vi "DeviceDiscover.vi"(0 "GenericDevice in":refnum<class "GenericDevice.lvclass">, 1 "Delay between send and receive [ms]":i32=5000, 5 "error in (no error)":errorcluster) -> (14 "GenericDevice out":refnum<class "GenericDevice.lvclass">, 15 "count":i32, 16 "ID":i32, 17 "returned command":string, 18 "error string (if existing)":string, 19 "error out":errorcluster)   [LabVIEW 2023, in "GenericDevice.lvclass"]
uses:
  GenericDevice.lvclass
  Discover.ctl
  GenericDevice.lvclass/GenericDevice.ctl
  f3c4c4a7-1197-4301-b128-d95ffad61759.vi
  8dcdfc4e-e41c-41c3-8bf5-06d7d5a87ca3.vi
  7995de1f-19cd-413c-9dd1-d9467f03dc24.vi
  <vilib>/JDP Science/JSONtext/Variant to JSON Text.vi
  <vilib>/JDP Science/JSONtext/Set Item.vi
  <vilib>/JDP Science/JSONtext/JSON text to Variant.vi
  <vilib>/JDP Science/JSONtext/LVClass Serializer/JSONtext LVClass Serializer.lvclass
panel:
  # "Connector Pane"
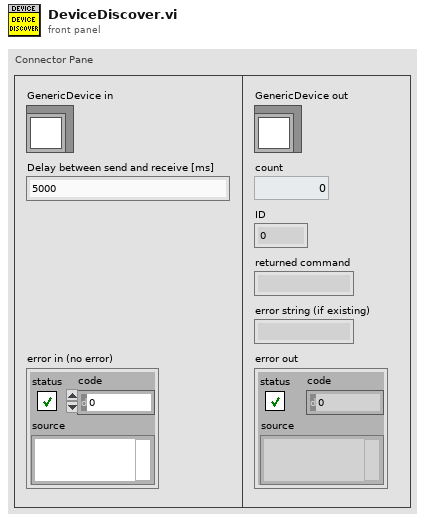
[diagram p1: front panel]
types:
  T1 = typedef "GenericDevice.lvclass/Discover.ctl" = cluster{"count":i32}
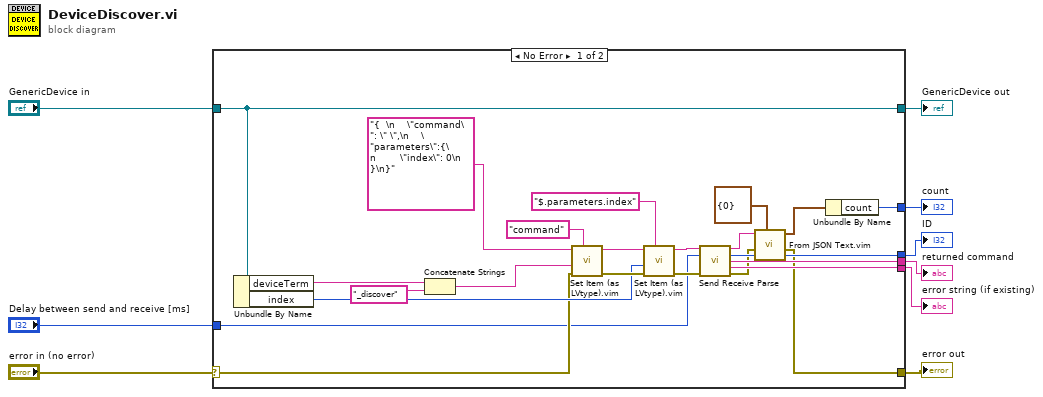
[diagram p0: block diagram]
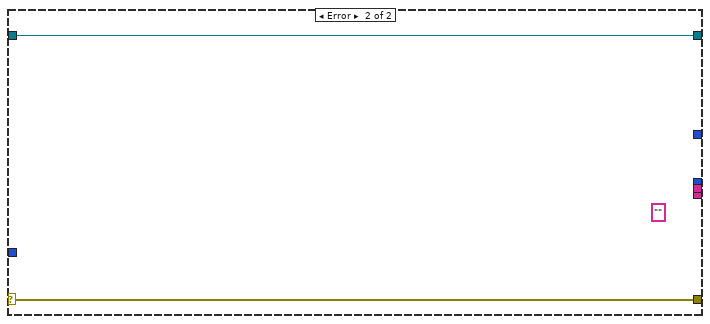
[diagram p2: hidden frame]
diagram:
  n1 = case shown="No Error" "error in (no error)" {
    selector: "error in (no error)" -> [w23 w34]
    tunnel: [w13 w34] -> w8
    tunnel: [w16 w33] -> w6
    tunnel: "GenericDevice in" -> [w16 w33]
    tunnel: [w11 _] -> w5
    tunnel: [w20 _] -> w4
    tunnel: [w19 _] -> w2
    tunnel: [w18 _] -> w3
    tunnel: "Delay between send and receive [ms]" -> [w10 _]
    frame No Error {
      n2 = Unbundle By Name(w16) -> ("deviceTerm"=w28:string, "index"=w24:i32)
      n3 = Concatenate Strings(w28, "_discover" ("string")) -> (w25:string)
      n4 = call "Set Item (as LVtype).vim"("$Path or Item Name"="command", "error in (no error)"=w23, "Anything"=w25, "JSON"="{  \n    \"command\": \" \",\n    \"parameters\":{\n        \"index\": 0\n    }\n}") -> ("error out"=w30:errorcluster, "<JSON>"=w31:string)  [unwired: 4 in, 1 out]
      n5 = call "Set Item (as LVtype).vim"("$Path or Item Name"="$.parameters.index", "error in (no error)"=w30, "Anything"=w24, "JSON"=w31) -> ("error out"=w21:errorcluster, "<JSON>"=w22:string)  [unwired: 4 in, 1 out]
      n6 = call "Send Receive Parse.vi"("<JSON>"=w22, "Delay between send and receive [ms]"=w10, "error in"=w21) -> ("results-JSON string"=w17:string, "ID"=w20:i32, "returned command"=w18:string, "error string (if existing)"=w19:string, "error out"=w14:errorcluster)  [unwired: 8 in]
      n7 = call "From JSON Text.vim"("Data Type and Default Value"=T1 {"count"=0} ("Chipsize"), "error in (no error)"=w14, "JSON"=w17) -> ("error out"=w13:errorcluster, "Data out"=w12:T1)  [unwired: 7 in]
      n8 = Unbundle By Name(w12) -> ("count"=w11:i32)
    }
    frame Error {
      (unwired) "" ("<JSON>")
    }
  }
  "error out" <- w8
  "GenericDevice out" <- w6
  "ID" <- w4
  "returned command" <- w3
  "error string (if existing)" <- w2
  "count" <- w5
